vi "WFStack2A.vi"(4 "error in (no error)":errorcluster, 6 "Waveform In 2":waveform(dbl)={"t0"=timestamp(0 s since 1904-01-01), "dt"=0.0, "Y"=[]}, 7 "Waveform In":waveform(dbl)={"t0"=timestamp(0 s since 1904-01-01), "dt"=0.0, "Y"=[]}) -> (0 "error out":errorcluster, 3 "Array":waveform(dbl)[](array[waveform]))   [LabVIEW 2013]
uses:
  <vilib>/Utility/error.llb/DialogType.ctl
  array/impl/ArrayLast_D.vi
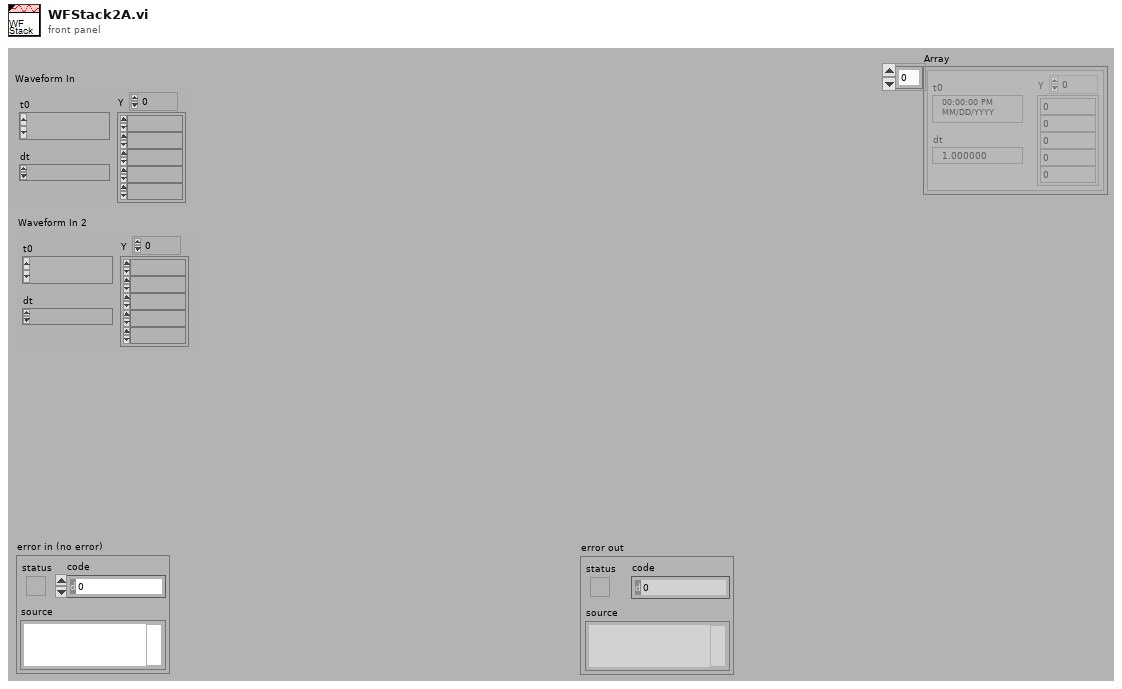
[diagram p1: front panel]
types:
  T1 = typedef "DialogType.ctl" = u16
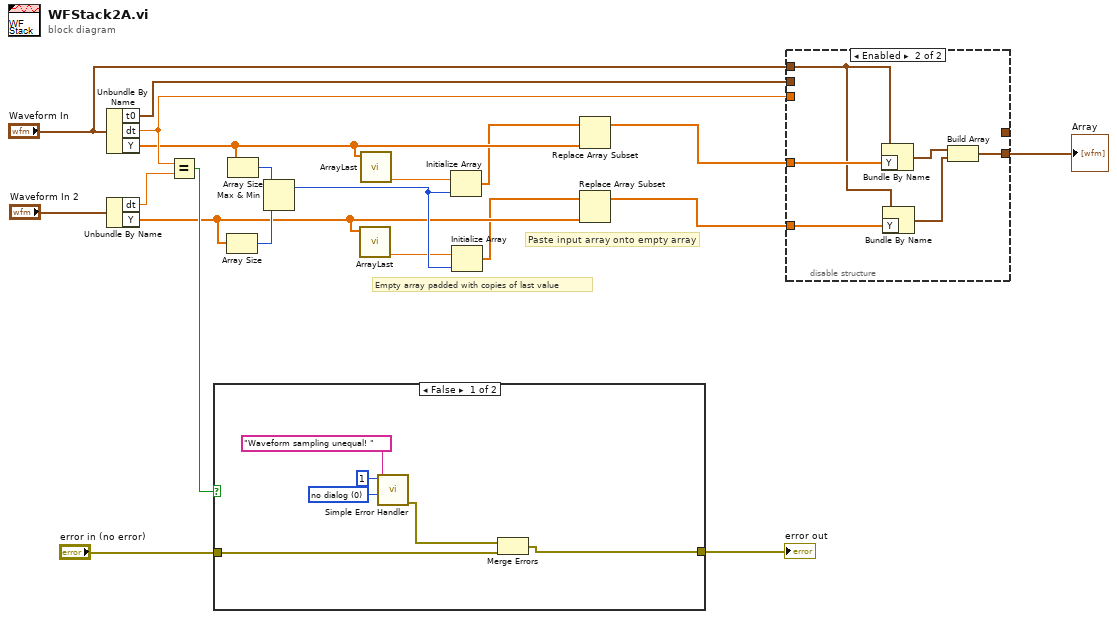
[diagram p0: block diagram]
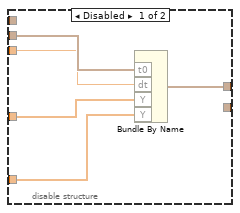
[diagram p2: hidden frame]
diagram:
  # "Paste input array onto empty array"
  # "Empty array padded with copies of last value"
  n1 = Unbundle By Name("Waveform In") -> ("t0"=w17:timestamp, "dt"=w16:dbl, "Y"=w3:dbl[])
  n2 = Unbundle By Name("Waveform In 2") -> ("dt"=w15:dbl, "Y"=w6:dbl[])
  n3 = Equal?(x=w16, y=w15) -> (x = y?=w20:bool)
  n4 = case shown="False" w20 {
    tunnel: [w25 w27] -> w18
    tunnel: "error in (no error)" -> [w26 w27]
    frame False {
      w22 = T1 0 items=["no dialog", "OK message", "continue or stop message", "OK message + warnings", "continue/stop + warnings"] ("type of dialog (OK msg:1)")
      n5 = call <vilib>:"Simple Error Handler.vi"("error code (no error:0)"=1, "error source (\" \")"="Waveform sampling unequal! " ("error source (\" \")"), "type of dialog (OK msg:1)"=w22) -> ("error out"=w24:errorcluster)  [unwired: 2 in, 4 out]
      n6 = Merge Errors(w24, w26) -> (w25:errorcluster)
    }
    frame True {
    }
  }
  "error out" <- w18
  n7 = Array Size(array=w6) -> (size(s)=w13:i32)
  n8 = Array Size(array=w3) -> (size(s)=w14:i32)
  n9 = Max & Min(x=w14, y=w13) -> (max(x,y)=w12:i32)  [unwired: 1 out]
  n10 = call-poly "ArrayLast.vi"("1D Array In"=w6) -> ("Last Element"=w5:dbl)  [unwired: 9 in, 1 out]
  n11 = call-poly "ArrayLast.vi"("1D Array In"=w3) -> ("Last Element"=w2:dbl)  [unwired: 9 in, 1 out]
  n12 = Initialize Array(w2, w12) -> (w1:dbl[])
  n13 = Initialize Array(w5, w12) -> (w4:dbl[])
  n14 = Replace Array Subset(array=w1, new element=w3) -> (w7:dbl[])  [unwired: 1 in]
  n15 = Replace Array Subset(array=w4, new element=w6) -> (w8:dbl[])  [unwired: 1 in]
  n16 = disable-structure shown="Enabled" {
    disable-tunnel: [w32 _] -> _
    disable-tunnel: w17 -> [w31 _]
    disable-tunnel: w16 -> [w30 _]
    disable-tunnel: w7 -> [w29 w38]
    disable-tunnel: w8 -> [w28 w37]
    disable-tunnel: "Waveform In" -> [_ w36]
    disable-tunnel: [_ w33] -> w9
    frame Disabled {
      n17 = Bundle By Name("t0"=w31, "dt"=w30, "Y"=w29, "Y"=w28) -> (w32:waveform(dbl))  [unwired: 1 in]
    }
    frame Enabled {
      n18 = Bundle By Name(cluster=w36, "Y"=w38) -> (w35:waveform(dbl))
      n19 = Bundle By Name(cluster=w36, "Y"=w37) -> (w34:waveform(dbl))
      n20 = Build Array(w35, w34) -> (w33:waveform(dbl)[])
    }
  }
  "Array" <- w9
